vi "Klinger ReadPosition.vi"(0 "Axe":u8(ring) items=["W", "X", "Y", "Z"], 2 "UnitDem":u8(ring)=2 caption="Unités" items=["Pas", "mm", "ps", "Degré (°)"], 3 "error in":errorcluster) -> (4 "PLimit":bool caption="Limite +", 5 "Moving":bool caption="Déplacement\nen cours", 6 "Position":dbl format="%#.1f", 7 "Statut":bool, 8 "NLimit":bool caption="Limite -", 9 "Cont Error":string caption="Message d'erreur", 10 "error out":errorcluster)   [LabVIEW 2010]
doc: "Ce VI retourne la position de l'axe moteur spécifié dans l'unité indiquée. Il retourne aussi l'état des interrupteurs de fin de course sur cet axe et indique si un déplacement y est en cours."
uses:
  <userlib>/Klinger/Klinger Lib.llb/Klinger ConvUnitSgl.vi
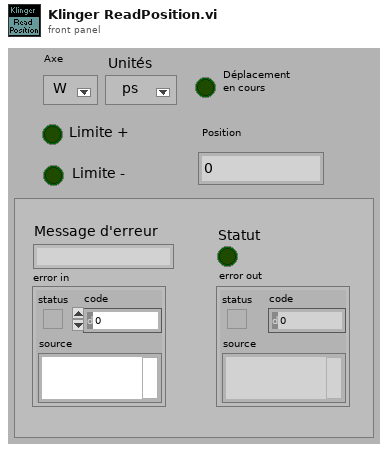
[diagram p1: front panel]
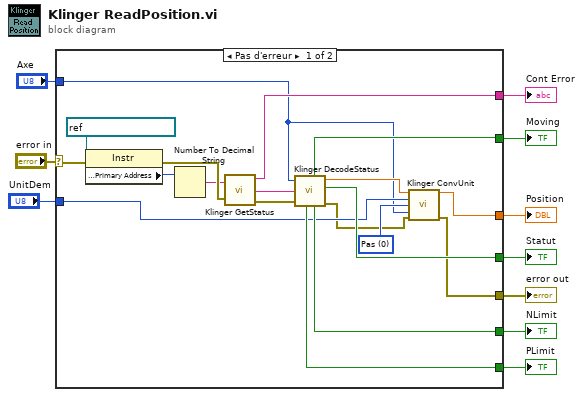
[diagram p0: block diagram]
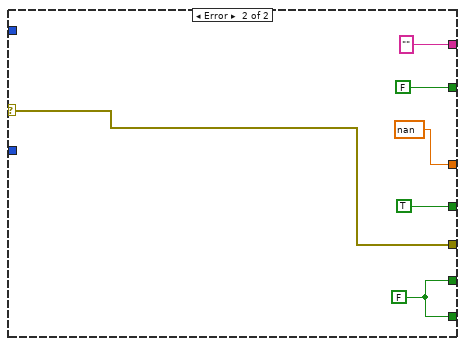
[diagram p2: hidden frame]
diagram:
  n1 = case shown="Pas d'erreur" "error in" {
    selector: "error in" -> [w27 w34]
    tunnel: [w21 w30] -> w10
    tunnel: [w22 w30] -> w9
    tunnel: [w14 nan] -> w8
    tunnel: "Axe" -> [w13 _]
    tunnel: [w11 w34] -> w6
    tunnel: [w18 "" ("Message D'erreur")] -> w5
    tunnel: [w23 TRUE ("Statut")] -> w4
    tunnel: [w20 FALSE] -> w2
    tunnel: "UnitDem" -> [w16 _]
    frame No Error {
      w17 = u8 0 items=["Pas", "mm", "ps"] ("UnitAct")
      n2 = property class="Instr"(reference=refnum<visa-resource-name> "GPIB0::6::INSTR", error in=w27) -> (error out=w26:errorcluster, "GPIB Settings:Primary Address"=w29:u16)  [unwired: 1 out]
      n3 = Number To Decimal String(number=w29) -> (decimal integer string=w24:string)  [unwired: 1 in]
      n4 = call <userlib>:"Klinger GetStatus.vi"("addresse"=w24, "error in"=w26) -> ("Message D'erreur"=w18:string, "Message Cont"=w25:string, "error out"=w19:errorcluster)  [unwired: 1 out]
      n5 = call <userlib>:"Klinger DecodeStatus.vi"("Axe"=w13, "Message Cont"=w25, "error in"=w19) -> ("PLimit"=w21:bool, "Moving"=w20:bool, "Position"=w15:dbl, "Statut"=w23:bool, "NLimit"=w22:bool, "error out"=w12:errorcluster)  [unwired: 2 in]
      n6 = call-poly <userlib>:"Klinger ConvUnit.vi"("ParamAct"=w15, "UnitDem"=w16, "UnitAct"=w17, "Axe"=w13, "error in"=w12) -> ("ParamDem"=w14:dbl, "error out"=w11:errorcluster)  [unwired: 9 in]
    }
    frame Error {
      w30 = FALSE
    }
  }
  "Moving" <- w2
  "PLimit" <- w10
  "NLimit" <- w9
  "Position" <- w8
  "Cont Error" <- w5
  "error out" <- w6
  "Statut" <- w4
